vi "nD Nonlinear System Solver (VI).vi"(5 "accuracy":dbl=1e-08 format="%0.2e", 6 "F(X)":T1, 7 "number of trials":u32=5, 8 "data":variant, 9 "End":dbl[](array[numeric]) format="%0.2f", 10 "Start":dbl[](array[numeric]) format="%0.2f", 11 "h":dbl=1e-08 format="%0.2e") -> (0 "error":i32, 1 "ticks":u32, 2 "f(Zeroes)":dbl[][](array[numeric]) format="%#.6g", 3 "Zeroes":dbl[][](array[numeric]) format="%#.6g")   [LabVIEW 2020, in "NI_Gmath.lvlib"]
doc: "Determines a set of solutions of a nonlinear system of equations in n dimensions beginning with a randomly chosen start point in n dimensions. You must manually select the polymorphic instance to use."
uses:
  NI_Gmath.lvlib
  functionRefnum nD.ctl
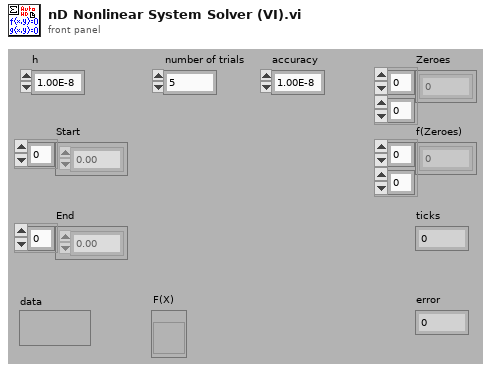
[diagram p1: front panel]
types:
  T1 = typedef "NI_Gmath.lvlib/functionRefnum nD.ctl" = refnum<vi>
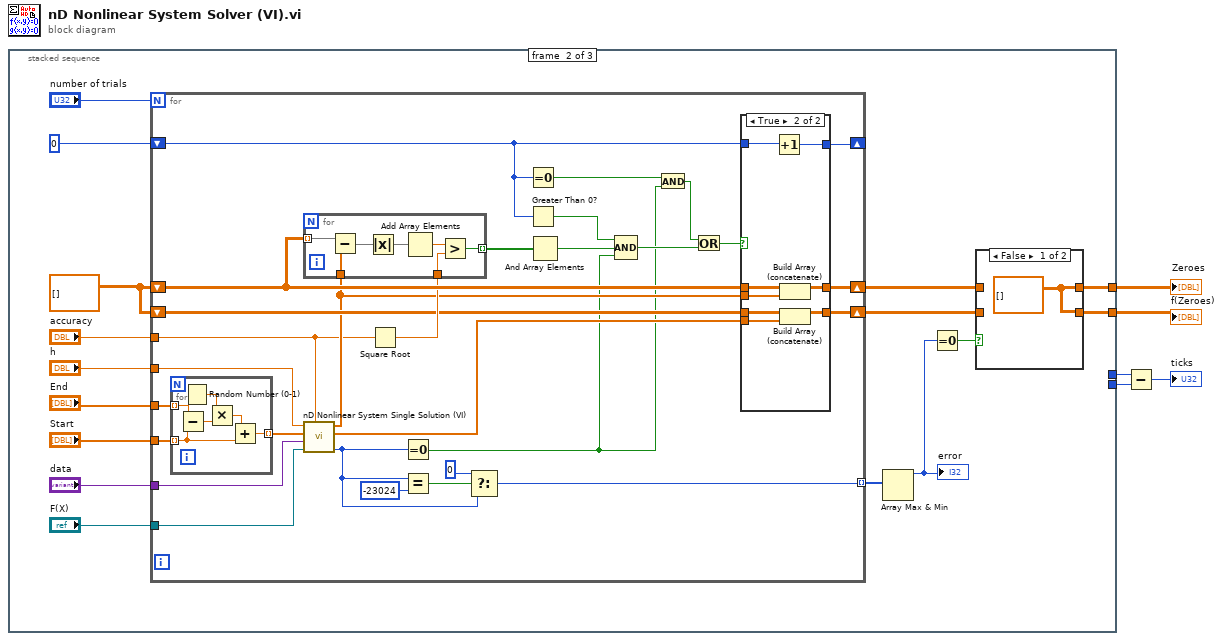
[diagram p0: block diagram]
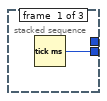
[diagram p2: hidden frame]
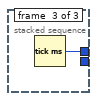
[diagram p5: hidden frame]
diagram:
  n1 = stacked-sequence {
    tunnel: [_ w21 _] -> w5
    tunnel: [_ w19 _] -> w4
    tunnel: [w6 _ _] -> w2
    tunnel: [_ _ w79] -> w3
    frame #0 {
      n2 = Tick Count (ms)() -> (millisecond timer value=w6:u32)
    }
    frame #1 {
      w8 = dbl[][] [] ("initialized array")
      n3 = for {
        N: "number of trials" -> [_]
        tunnel: "End" -> [w51]
        tunnel: "Start" -> [w50]
        shift-right: [w39] -> w20
        shift-left: w8 -> [w44]
        shift-right: [w40] -> w22
        shift-left: w8 -> [w49]
        tunnel: [w28] -> w13 mode=indexing
        shift-right: [w43] -> _
        shift-left: 0 -> [w36]
        tunnel: "accuracy" -> [w33]
        tunnel: "h" -> [w32]
        tunnel: "data" -> [w24]
        tunnel: "F(X)" -> [w23]
        n4 = for {
          tunnel: w51 -> [w75] mode=indexing
          tunnel: w50 -> [w73] mode=indexing
          tunnel: [w71] -> w46 mode=indexing
          n5 = Subtract(x=w75, y=w73) -> (x-y=w74:dbl)
          n6 = Random Number (0-1)() -> (number: 0 to 1=w70:dbl)
          n7 = Multiply(x=w70, y=w74) -> (x*y=w72:dbl)
          n8 = Add(x=w72, y=w73) -> (x+y=w71:dbl)
        }
        n9 = call "nD Nonlinear System Single Solution (VI).vi"("accuracy"=w33, "F(X)"=w23, "data"=w24, "Start"=w46, "h"=w32) -> ("error"=w29:i32, "f(Zeroes)"=w35:dbl[], "Zeroes"=w34:dbl[])  [unwired: 4 out]
        n10 = Square Root(x=w33) -> (sqrt(x)=w47:dbl)
        n11 = for {
          tunnel: w49 -> [w69] mode=indexing
          tunnel: w34 -> [w68]
          tunnel: [w64] -> w26 mode=indexing
          tunnel: w47 -> [w65]
          n12 = Subtract(x=w69, y=w68) -> (x-y=w67:dbl[])
          n13 = Absolute Value(x=w67) -> (abs(x)=w66:dbl[])
          n14 = Add Array Elements(numeric array=w66) -> (sum=w63:dbl)
          n15 = Greater?(x=w63, y=w65) -> (0:w64:bool)
        }
        n16 = Equal To 0?(x=w29) -> (x = 0?=w27:bool)
        n17 = Equal?(x=w29, y=-23024) -> (x = y?=w31:bool)
        n18 = Select(t=0, s=w31, f=w29) -> (s? t:f=w28:i32)
        n19 = Equal To 0?(x=w36) -> (x = 0?=w41:bool)
        n20 = Greater Than 0?(x=w36) -> (x > 0?=w38:bool)
        n21 = And Array Elements(Boolean array=w26) -> (logical AND=w25:bool)
        n22 = Compound Arithmetic op=AND(w38, w25, w27) -> (w37:bool)
        n23 = And(x=w41, y=w27) -> (x .and. y?=w42:bool)
        n24 = Or(x=w42, y=w37) -> (x .or. y?=w48:bool)
        n25 = case shown="True" w48 {
          tunnel: w44 -> [w54 w58]
          tunnel: [w54 w57] -> w39
          tunnel: w49 -> [w53 w61]
          tunnel: [w53 w60] -> w40
          tunnel: w34 -> [_ w62]
          tunnel: w35 -> [_ w59]
          tunnel: w36 -> [w52 w56]
          tunnel: [w52 w55] -> w43
          frame False {
          }
          frame True {
            n26 = Increment(x=w56) -> (x+1=w55:i32)
            n27 = Build Array (concatenate)(w61, w62) -> (w60:dbl[][])
            n28 = Build Array (concatenate)(w58, w59) -> (w57:dbl[][])
          }
        }
      }
      n29 = Array Max & Min(array=w13) -> (max value=w18:i32)  [unwired: 3 out]
      "error" <- w18
      n30 = Equal To 0?(x=w18) -> (x = 0?=w17:bool)
      n31 = case shown="False" w17 {
        tunnel: w22 -> [_ w78]
        tunnel: [w76 w78] -> w21
        tunnel: w20 -> [_ w77]
        tunnel: [w76 w77] -> w19
        frame False {
          w76 = dbl[][] [] ("initialized array")
        }
        frame True {
        }
      }
    }
    frame #2 {
      n32 = Tick Count (ms)() -> (millisecond timer value=w79:u32)
    }
  }
  "Zeroes" <- w5
  "f(Zeroes)" <- w4
  n33 = Subtract(x=w3, y=w2) -> (x-y=→"ticks":u32)
